vi "DSF.Engine.Memory.Index FIFO.Read.vi"(8 "error in (no error)":errorcluster, 9 "timeout in ms (0)":i32, 11 "Index FIFO in":refnum<class "DSF.Engine.Memory.Index FIFO.lvclass">) -> (0 "error out":errorcluster, 1 "timed out?":bool, 2 "index":i32, 3 "Index FIFO out":refnum<class "DSF.Engine.Memory.Index FIFO.lvclass">)   [LabVIEW 2016, in "DSF.Engine.lvlib" / "DSF.Engine.Memory.Index FIFO.lvclass"]
uses:
  DSF.Engine.Memory.Index FIFO.lvclass
  DSF.Engine.Memory.Index FIFO.lvclass/DSF.Engine.Memory.Index FIFO.ctl
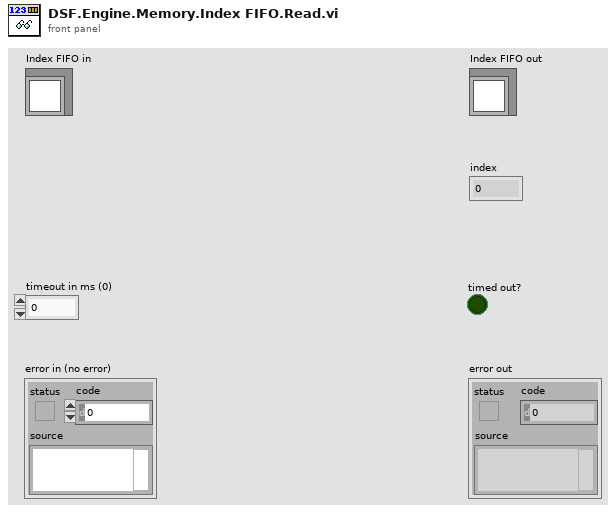
[diagram p1: front panel]
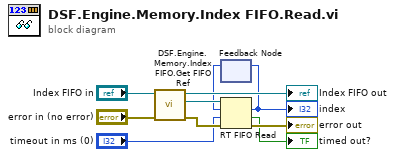
[diagram p0: block diagram]
diagram:
  n1 = call "DSF.Engine.Memory.Index FIFO.Get FIFO Ref.vi"("error in (no error)"="error in (no error)", "Index FIFO in"="Index FIFO in") -> ("error out"=w7:errorcluster, "FIFO"=w6:refnum<k33>, "Index FIFO out"=→"Index FIFO out":refnum<class "DSF.Engine.Memory.Index FIFO.lvclass">)  [unwired: 7 in]
  n2 = feedback #1() -> (w4:i32)  [unwired: 1 in]
  n3 = RT FIFO Read(0:w6, 1:w4, 2:"timeout in ms (0)", 3:w7) -> (9:w5:i32, 10:→"timed out?":bool, 11:→"error out":errorcluster)  [unwired: 2 out]
  "index" <- w5
  n4 = feedback-in #1(w5) -> ()
